vi "Parse JSON String.vi"(8 "error in (no error)":errorcluster, 10 "JSON String":string, 11 "Alpaca CLI Command Parser in":refnum<class "JSON Parser.lvclass">) -> (0 "error out":errorcluster, 2 "Value":variant, 3 "Alpaca CLI Command Parser out":refnum<class "JSON Parser.lvclass">)   [LabVIEW 2019, in "JKI JSON Serialization.lvlib" / "JSON Parser.lvclass"]
doc: "JKI JSON 1.1.10.37\nTomi Maila - JKI\nCopyright (c) 2017, JKI"
uses:
  JSON Parser.lvclass
  C:/Users/Patrick/Documents/GitHub/Instrument-Framework/lvsrc/SMOs/JSON-RPC-2019/lv-venv/lv.lib/vi.lib/addons/_JKI.lib/Serialization/JSON/Deserializer/Parser/Parser.lvclass
  Parser/Parser.lvclass/Parser.ctl
  JSON Parser.lvclass/JSON Parser.ctl
  JSON Lexer/JSON Lexer.lvclass
  C:/Users/Patrick/Documents/GitHub/Instrument-Framework/lvsrc/SMOs/JSON-RPC-2019/lv-venv/lv.lib/vi.lib/addons/_JKI.lib/Serialization/JSON/Deserializer/Lexer/Lexer.lvclass
  Parser/Parser.lvclass
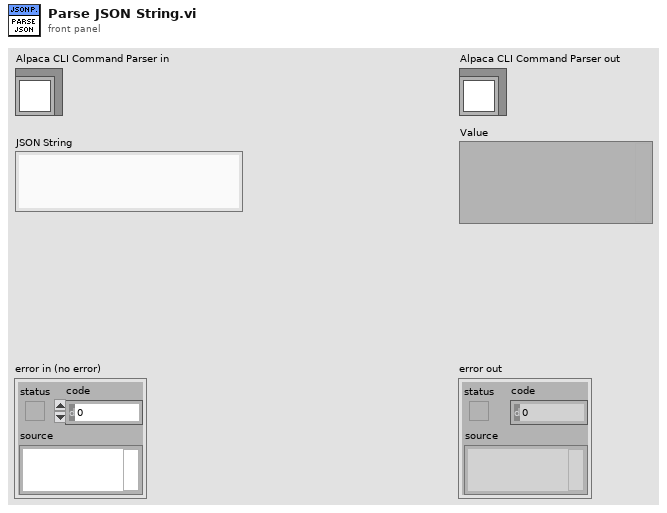
[diagram p1: front panel]
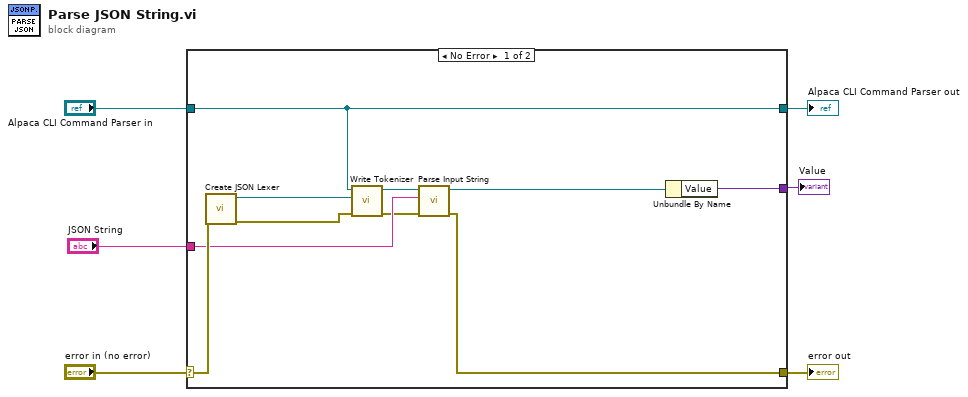
[diagram p0: block diagram]
diagram:
  n1 = case shown="No Error" "error in (no error)" {
    selector: "error in (no error)" -> [w16 w18]
    tunnel: [w15 w18] -> w5
    tunnel: [w11 w17] -> w3
    tunnel: "Alpaca CLI Command Parser in" -> [w11 w17]
    tunnel: "JSON String" -> [w12 _]
    tunnel: [w13 _] -> w1
    frame No Error {
      n2 = call "Create JSON Lexer.vi"("error in (no error)"=w16) -> ("error out"=w8:errorcluster, "JSON Lexer"=w7:refnum<class "JSON Lexer.lvclass">)  [unwired: 9 in]
      n3 = call "Write Tokenizer.vi"("error in (no error)"=w8, "Tokenizer"=w7, "Alpaca Parser in"=w11) -> ("error out"=w9:errorcluster, "Alpaca Parser out"=w10:refnum<class "JSON Parser.lvclass">)  [unwired: 7 in]
      n4 = call-dynamic "Parse Input String.vi"("error in (no error)"=w9, "String"=w12, "Alpaca Parser in"=w10) -> ("error out"=w15:errorcluster, "Alpaca Parser out"=w14:refnum<class "JSON Parser.lvclass">)  [unwired: 7 in]
      n5 = Unbundle By Name(w14) -> ("Value"=w13:variant)
    }
    frame Error {
    }
  }
  "error out" <- w5
  "Alpaca CLI Command Parser out" <- w3
  "Value" <- w1
